vi "Save Notes.vi"(0 "Filepath":path, 7 "Notes":string, 11 "Error In":errorcluster) -> (15 "Error Out":errorcluster)   [LabVIEW 2013]
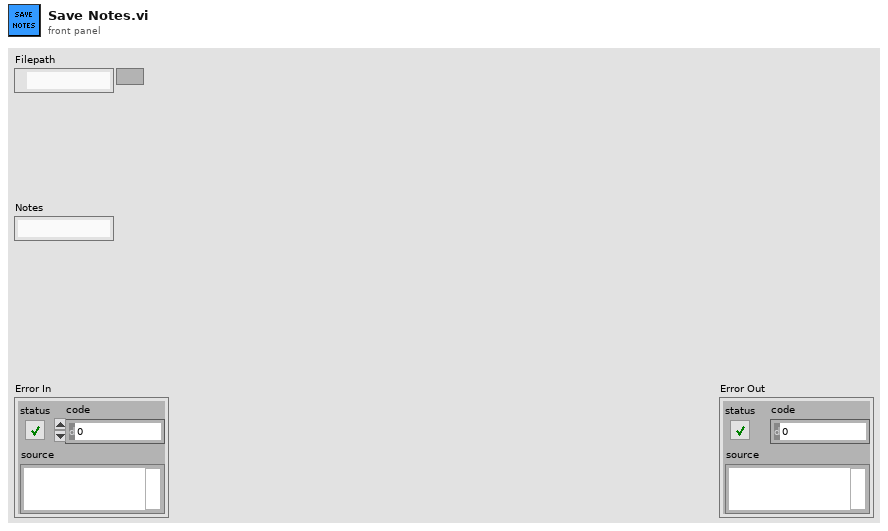
[diagram p1: front panel]
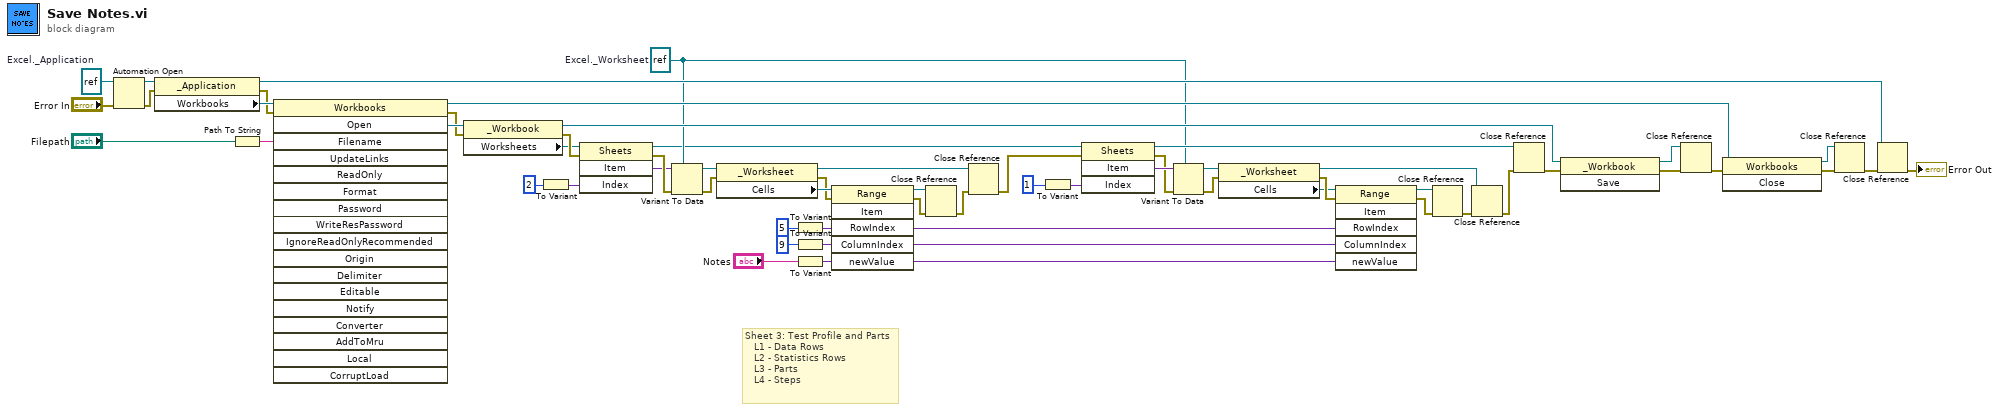
[diagram p0: block diagram]
diagram:
  w30 = refnum<k7> refnum  # Excel._Worksheet
  w55 = refnum<k7> refnum  # Excel._Application
  # "Sheet 3: Test Profile and Parts\n   L1 - Data Rows\n   L2 - Statistics Rows\n   L3 - Parts\n   L4 - Steps"
  n1 = Automation Open(error in (no error)="Error In", Automation Refnum=w55) -> (Automation Refnum=w56:refnum<k7>, error out=w57:errorcluster)  [unwired: 2 in]
  n2 = property class="_Application"(reference=w56, error in=w57) -> (reference out=w48:refnum<k7>, error out=w49:errorcluster, "Workbooks"=w58:refnum<k7>)
  n3 = Path To String(path="Filepath") -> (string=w45:string)
  n4 = invoke class="Workbooks" method="Open"(reference=w58, error in=w49, "Filename"=w45) -> (reference out=w52:refnum<k7>, error out=w47:errorcluster, "Open"=w54:refnum<k7>)  [unwired: 15 in, 15 out]
  n5 = property class="_Workbook"(reference=w54, error in=w47) -> (reference out=w41:refnum<k7>, error out=w33:errorcluster, "Worksheets"=w32:refnum<k7>)
  n6 = To Variant(anything=2) -> (Variant=w34:variant)
  n7 = invoke class="Sheets" method="Item"(reference=w32, error in=w33, "Index"=w34) -> (reference out=w27:refnum<k7>, error out=w36:errorcluster, "Item"=w35:variant)  [unwired: 1 in, 1 out]
  n8 = Variant To Data(error in=w36, type=w30, Variant=w35) -> (data=w37:refnum<k7>, error out=w38:errorcluster)
  n9 = property class="_Worksheet"(reference=w37, error in=w38) -> (reference out=w26:refnum<k7>, error out=w11:errorcluster, "Cells"=w12:refnum<k7>)
  n10 = To Variant(anything=5) -> (Variant=w6:variant)
  n11 = To Variant(anything=9) -> (Variant=w5:variant)
  n12 = To Variant(anything="Notes") -> (Variant=w4:variant)
  n13 = invoke class="Range" method="Item"(reference=w12, error in=w11, "RowIndex"=w6, "ColumnIndex"=w5, "newValue"=w4) -> (reference out=w10:refnum<k7>, error out=w9:errorcluster)  [unwired: 1 in, 4 out]
  n14 = Close Reference(reference=w10, error in (no error)=w9) -> (error out=w25:errorcluster)
  n15 = Close Reference(reference=w26, error in (no error)=w25) -> (error out=w24:errorcluster)
  n16 = To Variant(anything=1) -> (Variant=w20:variant)
  n17 = invoke class="Sheets" method="Item"(reference=w27, error in=w24, "Index"=w20) -> (reference out=w39:refnum<k7>, error out=w18:errorcluster, "Item"=w19:variant)  [unwired: 1 in, 1 out]
  n18 = Variant To Data(error in=w18, type=w30, Variant=w19) -> (data=w17:refnum<k7>, error out=w16:errorcluster)
  n19 = property class="_Worksheet"(reference=w17, error in=w16) -> (reference out=w14:refnum<k7>, error out=w8:errorcluster, "Cells"=w7:refnum<k7>)
  n20 = invoke class="Range" method="Item"(reference=w7, error in=w8, "RowIndex"=w6, "ColumnIndex"=w5, "newValue"=w4) -> (reference out=w3:refnum<k7>, error out=w2:errorcluster)  [unwired: 1 in, 4 out]
  n21 = Close Reference(reference=w3, error in (no error)=w2) -> (error out=w15:errorcluster)
  n22 = Close Reference(reference=w14, error in (no error)=w15) -> (error out=w40:errorcluster)
  n23 = Close Reference(reference=w39, error in (no error)=w40) -> (error out=w46:errorcluster)
  n24 = invoke class="_Workbook" method="Save"(reference=w41, error in=w46) -> (reference out=w42:refnum<k7>, error out=w43:errorcluster)  [unwired: 1 in, 1 out]
  n25 = Close Reference(reference=w42, error in (no error)=w43) -> (error out=w44:errorcluster)
  n26 = invoke class="Workbooks" method="Close"(reference=w52, error in=w44) -> (reference out=w51:refnum<k7>, error out=w50:errorcluster)  [unwired: 1 in, 1 out]
  n27 = Close Reference(reference=w51, error in (no error)=w50) -> (error out=w53:errorcluster)
  n28 = Close Reference(reference=w48, error in (no error)=w53) -> (error out=→"Error Out":errorcluster)
